vi "get_by_asset.path.vi"() -> (2 "path":string)   [LabVIEW 2020, in "asset.lvclass"]
uses:
  Run/Run.lvclass/Run.ctl
  asset.lvclass
  asset.lvclass/asset.ctl
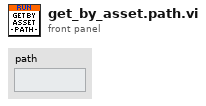
[diagram p1: front panel]
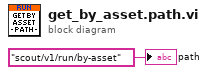
[diagram p0: block diagram]
diagram:
  "path" <- "scout/v1/run/by-asset"
